vi "Add MsgQ.vi"(8 "error in (no error)":errorcluster, 11 "MsgQ Name":string) -> (0 "error out":errorcluster, 3 "Added?":bool)   [LabVIEW 2009, in "Interloop MessageQ.lvlib"]
doc: "Adds a message to the global message queue manager. Requires a message Queue name."
uses:
  Interloop MessageQ.lvlib
  Message queue handler mode enums.ctl
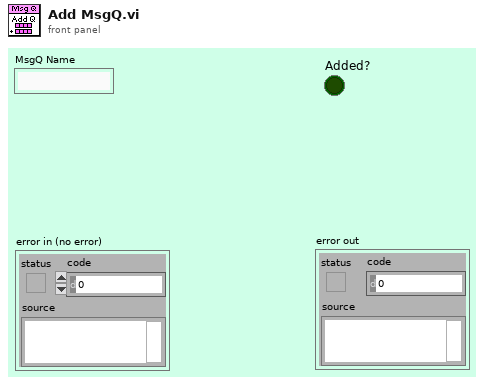
[diagram p1: front panel]
types:
  T1 = typedef "Interloop MessageQ.lvlib/Message queue handler mode enums.ctl" = enum16{"Initialize", "Create MsgQ", "Destroy MsgQ", "Send Message", "Broadcast Message", "Read Message", "Close"}
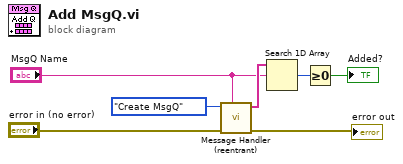
[diagram p0: block diagram]
diagram:
  n1 = call "Message Handler (reentrant).vi"("MsgQ Name"="MsgQ Name", "error in (no error)"="error in (no error)", "Mode"=Message_queue_handler_mode_enums."Create MsgQ") -> ("error out"=→"error out":errorcluster, "Queue Names"=w4:string[])  [unwired: 1 in, 6 out]
  n2 = Search 1D Array(1D array=w4, element="MsgQ Name") -> (index of element=w2:i32)  [unwired: 1 out]
  n3 = Greater Or Equal To 0?(x=w2) -> (x >= 0?=→"Added?":bool)
